vi "Plot Meas channels.vi"() -> ()   [LabVIEW 2022 SP3]
uses:
  Anemometry Sub Vis/Controls/Data for Inst Type.ctl
  Anemometry Sub Vis/Globals/Meas_global.vi
panel:
  in  "Number of Series":i32=1 min=1
  in  "Mode":T1
  in  "stop":bool
  in  "Plots":u16[](array[ring])=[4, 71, 140, 237, 267, 329, 404, 466] items=["None", "RZ (C0_P00)", "RZ (C0_P01)", "RZ (C0_P02)", "RZ (C0_P03)", "RZ (C0_P04)", "RZ (C0_P05)", "RZ (C0_P06)", "RZ (C0_P07)", "RZ (C0_P10)", "RZ (C0_P11)", "RZ (C0_P12)", "RZ (C0_P13)", "RZ (C0_P14)", "RZ (C0_P15)", "RZ (C0_P16)", "RZ (C0_P17)", "RZ (C0_P20)", "RZ (C0_P21)", "RZ (C0_P22)", "RZ (C0_P23)", "RZ (C0_P24)", "RZ (C0_P25)", "RZ (C0_P26)", "RZ (C0_P27)", "RZ (C0_P30)", "RZ (C0_P31)", "RZ (C0_P32)", "RZ (C0_P33)", "RZ (C0_P34)", "RZ (C0_P35)", "RZ (C0_P36)", "RZ (C0_P37)", "RZ (C0_P40)", "RZ (C0_P41)", "RZ (C0_P42)", "RZ (C0_P43)", "RZ (C0_P44)", "RZ (C0_P45)", "RZ (C0_P46)", "RZ (C0_P47)", "RZ (C0_P50)", "RZ (C0_P51)", "RZ (C1_P73)", "RZ (C0_P53)", "RZ (C0_P54)", "RZ (C0_P55)", "RZ (C0_P56)", "RZ (C0_P57)", "RZ (C0_P60)", "RZ (C0_P62)", "RZ (C0_P63)", "RZ (C0_P64)", "RZ (C0_P65)", "RZ (C0_P66)", "RZ (C0_P67)", "RZ (C0_P70)", "RZ (C0_P71)", "RZ (C0_P72)", "RZ (C0_P73)", "RZ (C0_P74)", "RZ (C0_P75)", "RZ (C0_P76)", "RZ (C0_P77)", "RZ (C1_P00)", "RZ (C1_P01)", "RZ (C1_P02)", "RZ (C1_P03)", "RZ (C1_P04)", "RZ (C1_P05)", "RZ (C1_P06)", "RZ (C1_P07)", "RZ (C1_P10)", "RZ (C1_P11)", "RZ (C1_P12)", "RZ (C1_P13)", "RZ (C1_P14)", "RZ (C1_P15)", "RZ (C1_P16)", "RZ (C1_P17)", "RZ (C1_P20)", "RZ (C1_P21)", "RZ (C1_P22)", "RZ (C1_P23)", "RZ (C1_P24)", "RZ (C1_P25)", "RZ (C1_P26)", "RZ (C1_P27)", "RZ (C1_P30)", "RZ (C1_P31)", "RZ (C1_P32)", "RZ (C1_P33)", "RZ (C1_P34)", "RZ (C1_P35)", "RZ (C1_P36)", "RZ (C1_P37)", "RZ (C1_P40)", "RZ (C1_P41)", "RZ (C1_P42)", "RZ (C1_P43)", "RZ (C1_P44)", "RZ (C1_P45)", "RZ (C1_P46)", "RZ (C1_P47)", "RZ (C1_P50)", "RZ (C1_P51)", "RZ (C1_P52)", "RZ (C1_P53)", "RZ (C1_P54)", "RZ (C1_P55)", "RZ (C1_P56)", "RZ (C1_P57)", "RZ (C1_P60)", "RZ (C1_P61)", "RZ (C1_P62)", "RZ (C1_P63)", "RZ (C2_P00)", "RZ (C2_P01)", "RZ (C2_P02)", "RZ (C2_P03)", "RZ (C2_P04)", "RZ (C2_P05)", "RZ (C2_P06)", "RZ (C2_P07)", "RZ (C2_P10)", "RZ (C2_P11)", "RZ (C2_P12)", "RZ (C2_P13)", "RZ (C2_P14)", "RZ (C2_P15)", "RZ (C2_P16)", "RZ (C2_P17)", "RZ (C2_P20)", "RZ (C2_P21)", "RZ (C2_P22)", "RZ (C2_P23)", "RZ (C2_P24)", "RZ (C2_P25)", "RZ (C2_P26)", "RZ (C2_P27)", "RZ (C2_P31)", "RZ (C2_P32)", "RZ (C2_P33)", "RZ (C2_P34)", "RZ (C2_P35)", "RZ (C2_P36)", "RZ (C2_P37)", "RZ (C2_P40)", "RZ (C2_P41)", "RZ (C2_P42)", "RZ (C2_P43)", "RZ (C2_P44)", "RZ (C2_P45)", "RZ (C2_P46)", "RZ (C2_P47)", "RZ (C2_P50)", "RZ (C2_P51)", "RZ (C2_P52)", "RZ (C2_P53)", "RZ (C2_P54)", "RZ (C2_P55)", "RZ (C2_P56)", "RZ (C2_P57)", "RZ (C2_P60)", "RZ (C2_P61)", "RZ (C2_P62)", "RZ (C2_P63)", "RZ (C2_P64)", "RZ (C2_P65)", "RZ (C2_P66)", "RZ (C2_P67)", "RZ (C2_P70)", "RZ (C2_P71)", "RZ (C2_P72)", "RZ (C2_P73)", "RZ (C2_P74)", "RZ (C2_P75)", "RZ (C2_P76)", "RZ (C2_P77)", "RZ (C3_P00)", "RZ (C3_P01)", "RZ (C3_P02)", "RZ (C3_P03)", "RZ (C3_P04)", "RZ (C3_P05)", "RZ (C3_P06)", "RZ (C3_P07)", "RZ (C3_P10)", "RZ (C3_P11)", "RZ (C3_P12)", "RZ (C3_P13)", "RZ (C3_P14)", "RZ (C3_P15)", "RZ (C3_P16)", "RZ (C3_P17)", "RZ (C3_P20)", "RZ (C3_P21)", "RZ (C3_P22)", "RZ (C3_P23)", "RZ (C3_P24)", "RZ (C3_P25)", "RZ (C3_P26)", "RZ (C3_P27)", "RZ (C3_P30)", "RZ (C3_P31)", "RZ (C3_P33)", "RZ (C3_P34)", "RZ (C3_P35)", "RZ (C3_P36)", "RZ (C3_P37)", "RZ (C3_P40)", "RZ (C3_P41)", "RZ (C3_P42)", "RZ (C3_P43)", "RZ (C3_P44)", "RZ (C3_P45)", "RZ (C3_P46)", "RZ (C3_P47)", "RZ (C3_P50)", "RZ (C3_P51)", "RZ (C3_P52)", "RZ (C3_P53)", "RZ (C3_P54)", "RZ (C3_P55)", "RZ (C3_P56)", "RZ (C3_P60)", "RZ (C3_P61)", "RZ (C3_P62)", "RZ (C3_P63)", "RZ (C3_P64)", "RZ (C3_P65)", "RZ (C3_P66)", "RZ (C3_P70)", "RZ (C3_P71)", "RZ (C3_P72)", "RZ (C3_P73)", "RZ (C3_P74)", "RZ (C3_P75)", "RZ (C3_P77)", "RZ (C4_P00)", "RZ (C4_P01)", "RZ (C4_P02)", "RZ (C4_P03)", "RZ (C4_P04)", "RZ (C4_P05)", "RZ (C4_P06)", "RZ (C4_P07)", "RZ (C4_P10)", "RZ (C4_P11)", "RZ (C4_P12)", "RZ (C4_P13)", "RZ (C4_P15)", "RZ (C4_P16)", "RZ (C4_P17)", "RZ (C4_P20)", "RZ (C4_P21)", "RZ (C4_P22)", "RZ (C4_P23)", "RZ (C4_P24)", "RZ (C4_P26)", "RZ (C4_P27)", "RZ (C4_P30)", "RZ (C4_P32)", "RZ (C4_P33)", "RZ (C4_P34)", "RZ (C4_P35)", "RZ (C4_P36)", "RZ (C4_P37)", "RZ (C4_P40)", "RZ (C4_P41)", "RZ (C4_P42)", "RZ (C4_P43)", "RZ (C4_P44)", "RZ (C4_P45)", "RZ (C4_P46)", "RZ (C4_P47)", "RZ (C4_P50)", "RZ (C4_P51)", "RZ (C4_P52)", "RZ (C4_P53)", "RZ (C4_P54)", "RZ (C4_P55)", "RZ (C4_P56)", "RZ (C4_P57)", "RZ (C4_P60)", "RZ (C4_P61)", "RZ (C4_P62)", "RZ (C4_P63)", "RZ (C4_P64)", "RZ (C4_P65)", "RZ (C4_P66)", "RZ (C4_P67)", "RZ (C4_P70)", "RZ (C4_P71)", "RZ (C4_P72)", "RZ (C4_P73)", "RZ (C4_P74)", "RZ (C4_P75)", "RZ (C4_P76)", "RZ (C4_P77)", "RZ (C5_P00)", "RZ (C5_P01)", "RZ (C5_P02)", "RZ (C5_P03)", "RZ (C5_P04)", "RZ (C5_P05)", "RZ (C5_P06)", "RZ (C5_P07)", "RZ (C5_P10)", "RZ (C5_P11)", "RZ (C5_P12)", "RZ (C5_P13)", "RZ (C5_P14)", "RZ (C5_P15)", "RZ (C5_P16)", "RZ (C5_P17)", "RZ (C5_P20)", "RZ (C5_P21)", "RZ (C5_P22)", "RZ (C5_P23)", "RZ (C5_P24)", "RZ (C5_P25)", "RZ (C5_P26)", "RZ (C5_P27)", "RZ (C5_P30)", "RZ (C5_P31)", "RZ (C5_P32)", "RZ (C5_P33)", "RZ (C5_P34)", "RZ (C5_P35)", "RZ (C5_P36)", "RZ (C5_P37)", "RZ (C5_P40)", "RZ (C5_P41)", "RZ (C5_P42)", "RZ (C5_P43)", "RZ (C5_P44)", "RZ (C5_P45)", "RZ (C5_P46)", "RZ (C5_P47)", "RZ (C5_P50)", "RZ (C5_P51)", "RZ (C5_P52)", "RZ (C5_P53)", "RZ (C5_P54)", "RZ (C5_P55)", "RZ (C5_P56)", "RZ (C5_P60)", "RZ (C5_P61)", "RZ (C5_P62)", "RZ (C5_P63)", "RZ (C5_P64)", "RZ (C5_P65)", "RZ (C5_P66)", "RZ (C5_P67)", "RZ (C5_P71)", "RZ (C5_P72)", "RZ (C5_P73)", "RZ (C5_P74)", "RZ (C5_P75)", "RZ (C5_P76)", "RZ (C5_P77)", "RZ (C6_P02)", "RZ (C6_P03)", "RZ (C6_P04)", "RZ (C6_P05)", "RZ (C6_P06)", "RZ (C6_P07)", "RZ (C6_P12)", "RZ (C6_P13)", "RZ (C6_P14)", "RZ (C6_P15)", "RZ (C6_P16)", "RZ (C6_P17)", "RZ (C6_P20)", "RZ (C6_P21)", "RZ (C6_P22)", "RZ (C6_P23)", "RZ (C6_P24)", "RZ (C6_P25)", "RZ (C6_P26)", "RZ (C6_P27)", "RZ (C6_P30)", "RZ (C6_P31)", "RZ (C6_P32)", "RZ (C6_P33)", "RZ (C6_P34)", "RZ (C6_P35)", "RZ (C6_P36)", "RZ (C6_P37)", "RZ (C6_P40)", "RZ (C6_P41)", "RZ (C6_P42)", "RZ (C6_P43)", "RZ (C6_P44)", "RZ (C6_P45)", "RZ (C6_P46)", "RZ (C6_P47)", "RZ (C6_P50)", "RZ (C6_P51)", "RZ (C6_P52)", "RZ (C6_P53)", "RZ (C6_P54)", "RZ (C6_P55)", "RZ (C6_P56)", "RZ (C6_P60)", "RZ (C6_P61)", "RZ (C6_P62)", "RZ (C6_P63)", "RZ (C6_P64)", "RZ (C6_P65)", "RZ (C6_P66)", "RZ (C6_P67)", "RZ (C6_P70)", "RZ (C6_P71)", "RZ (C6_P72)", "RZ (C6_P73)", "RZ (C6_P74)", "RZ (C6_P75)", "RZ (C6_P76)", "RZ (C6_P77)", "RZ (C7_P00)", "RZ (C7_P01)", "RZ (C7_P02)", "RZ (C7_P03)", "RZ (C7_P04)", "RZ (C7_P05)", "RZ (C7_P06)", "RZ (C7_P07)", "RZ (C7_P10)", "RZ (C7_P11)", "RZ (C7_P12)", "RZ (C7_P13)", "RZ (C7_P14)", "RZ (C7_P15)", "RZ (C7_P16)", "RZ (C7_P17)", "RZ (C7_P20)", "RZ (C7_P21)", "RZ (C7_P22)", "RZ (C7_P23)", "RZ (C7_P24)", "RZ (C7_P25)", "RZ (C7_P26)", "RZ (C7_P27)", "RZ (C7_P30)", "RZ (C7_P31)", "RZ (C7_P32)", "RZ (C7_P33)", "RZ (C7_P34)", "RZ (C7_P35)", "RZ (C7_P36)", "RZ (C7_P37)", "RZ (C7_P40)", "RZ (C7_P41)", "RZ (C7_P42)", "RZ (C7_P43)", "RZ (C7_P44)", "RZ (C7_P45)", "RZ (C7_P46)", "RZ (C7_P47)", "RZ (C7_P50)", "RZ (C7_P51)", "RZ (C7_P52)", "RZ (C7_P53)", "RZ (C7_P54)", "RZ (C7_P55)", "RZ (C7_P56)", "RZ (C7_P57)", "RZ (C7_P60)", "RZ (C7_P61)", "RZ (C7_P62)", "RZ (C7_P63)", "RZ (C7_P64)", "RZ (C7_P65)", "RZ (C7_P66)", "RZ (C7_P67)", "RZ (C7_P70)", "RZ (C7_P71)", "RZ (C7_P72)", "RZ (C7_P73)", "RZ (C7_P74)", "RZ (C7_P75)", "RZ (C7_P76)", "RZ (C7_P77)", "FF (C)", "FF (Cref)"]
  out "XY Graph":cluster{"Time (s)":dbl[], "Eng Values":dbl[]}[](graph)
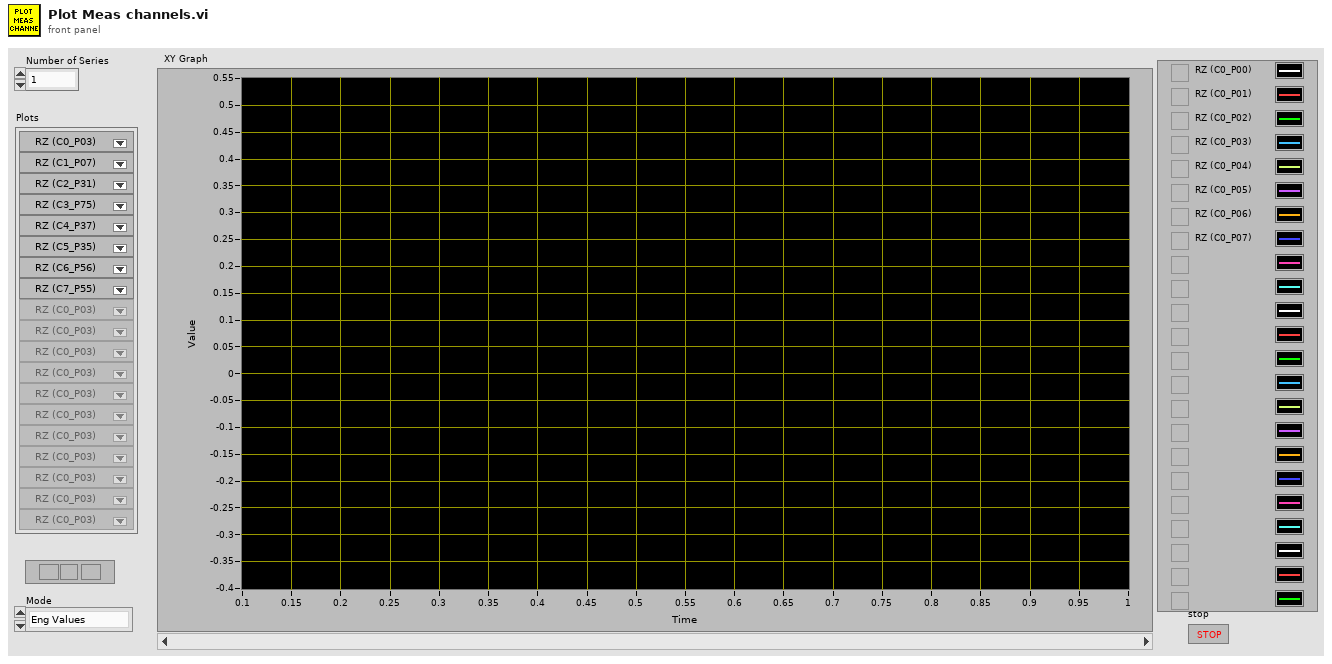
[diagram p1: front panel]
types:
  T1 = typedef "Data for Inst Type.ctl" = enum16{"Eng Values", "Voltage"}
  T2 = typedef "Analysis_info_cluster.ctl" = cluster{"Colour":u32, "Inst type":T3, "Inst name":string, "Symbol":string, "Code name":string, "Extra Info":string, "Inst Array":T4, "Extra Titles":string[], "Extra Values":string[], "U":dbl, "u^2":dbl, "u^3":dbl, "u^4":dbl, "Skew_u":dbl, "Kurt_u":dbl, "Sd Error in Mean":dbl, "% u'/U":dbl, "X":dbl, "Y":dbl, "Z":dbl, "Timescale integral Estimate":dbl, "Sd Error in Variance":dbl, "Calib File":path, "Calib Constants":dbl[], "Output Position":bool, "Stats":enum16{"None", "Basic", "Full"}, "Av Sampling Rate":dbl, "Av No of Samples":dbl, "Total Meas Time (s)":dbl, "ADAM Ch Name":string, "Max value":dbl, "Min value":dbl, "Req Sample Rate Hz":dbl, "Sync Delay Time (s)":dbl, "Ch No":i16, "Device":string, "Use Latest Calib":bool, "Port":string, "Metadata Ch Names":string[], "Metadata Ch Values":string[], "Label":string}
  T3 = typedef "Inst_type.ctl" = enum16{"Raw voltage", "Raw with zero offsetting", "Propeller anemometer", "Pressure Transducer", "Pitot-static tube", "Hot wire", "Cross wire 1", "Cross wire 2", "Generic Linear", "Generic Polynomial", "Generic BackPoly", "Fast FID", "Thermocouple", "Cold wire", "Pulsed Wire", "LDA Vel", "LDA Tran time", "LDA Arr time", "Microphone"}
  T4 = typedef "Instrument_Array.ctl" = enum16{"PWA", "LDA", "Analogue"}
  T5 = typedef "Time_Trace_Cluster.ctl" = cluster{"Weighting":dbl[], "Voltage":dbl[], "Eng Values":dbl[]}
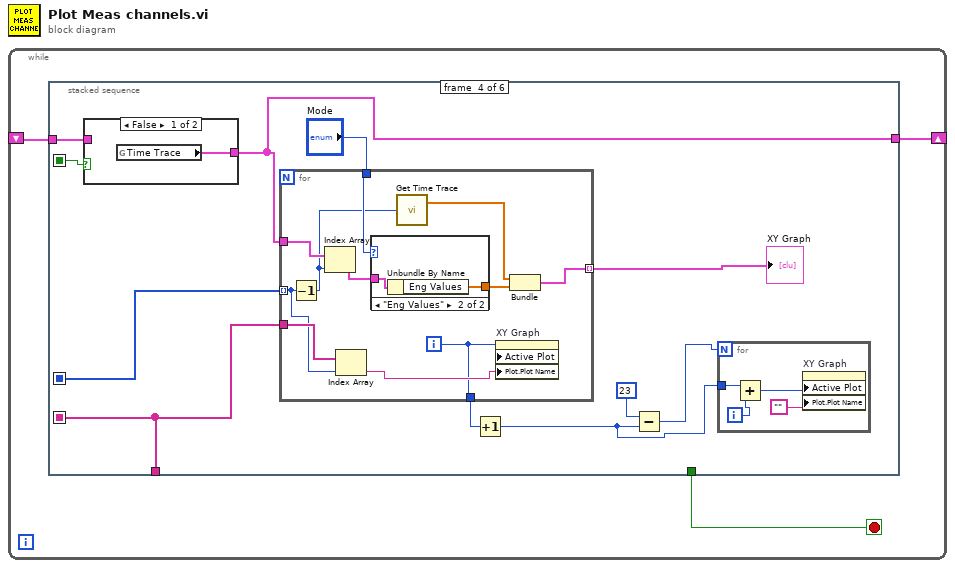
[diagram p0: block diagram]
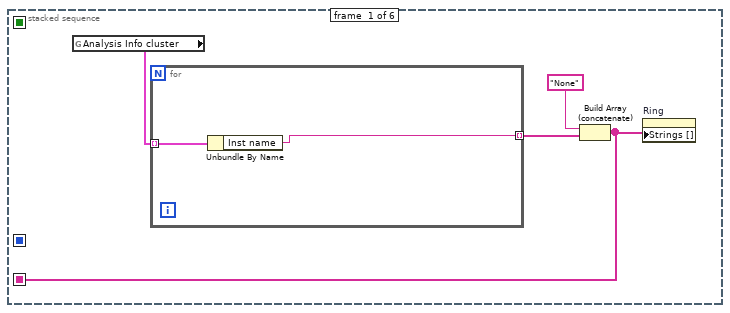
[diagram p2: hidden frame]
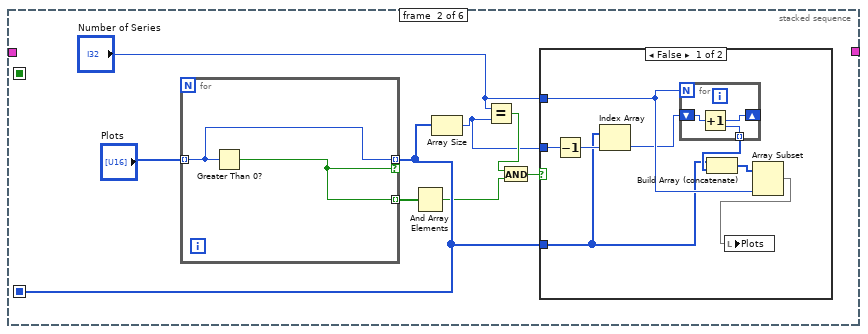
[diagram p3: hidden frame]
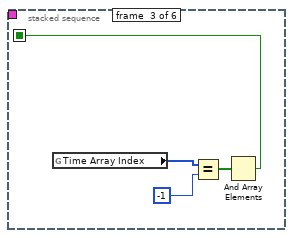
[diagram p5: hidden frame]
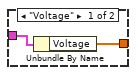
[diagram p7: hidden frame]
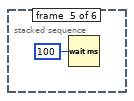
[diagram p8: hidden frame]
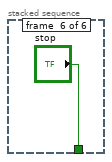
[diagram p9: hidden frame]
diagram:
  n1 = while {
    shift-right: [w2] -> _
    shift-left: _ -> [w1]
    stop <- w3 stop-if-true
    n2 = stacked-sequence {
      seq-local: [_ w15 _ _ _ _] -> [_ _ _ w43 _ _]
      seq-local: [w4 _ _ _ _ _] -> [_ _ _ w38 _ _]
      seq-local: [_ _ w30 _ _ _] -> [_ _ _ w36 _ _]
      tunnel: [_ _ _ w38 _ _] -> _
      tunnel: [_ _ _ _ _ "stop"] -> w3
      tunnel: [_ _ _ w35 _ _] -> w2
      tunnel: w1 -> [_ _ _ w34 _ _]
      frame #0 {
        n3 = global read "Meas_global.vi" "Analysis Info cluster"() -> (w5:T2[])
        n4 = for {
          tunnel: w5 -> [w9] mode=indexing
          tunnel: [w8] -> w7 mode=indexing
          n5 = Unbundle By Name(w9) -> ("Inst name"=w8:string)
        }
        n6 = Build Array (concatenate)("None", w7) -> (w4:string[])
        n7 = property on="Ring" class="Ring (strict)"("Strings []"=w4) -> ()  [unwired: 2 in, 2 out]
      }
      frame #1 {
        n8 = for {
          tunnel: "Plots" -> [w29] mode=indexing
          tunnel: [w29] -> w15 mode=indexing if=w28
          tunnel: [w28] -> w16 mode=indexing
          n9 = Greater Than 0?(x=w29) -> (x > 0?=w28:bool)
        }
        n10 = And Array Elements(Boolean array=w16) -> (logical AND=w13:bool)
        n11 = Array Size(array=w15) -> (size(s)=w10:i32)
        n12 = Equal?(x="Number of Series", y=w10) -> (x = y?=w14:bool)
        n13 = And(x=w14, y=w13) -> (x .and. y?=w12:bool)
        n14 = case shown="False" w12 {
          tunnel: w15 -> [w19 _]
          tunnel: "Number of Series" -> [w22 _]
          tunnel: w10 -> [w21 _]
          frame False {
            n15 = Decrement(x=w21) -> (x-1=w20:i32)
            n16 = Index Array(array=w19, index=w20) -> (element=w18:u16)
            n17 = for {
              N: w22 -> [_]
              tunnel: [w26] -> w23 mode=indexing
              shift-right: [w26] -> _
              shift-left: w18 -> [w27]
              n18 = Increment(x=w27) -> (x+1=w26:u16)
            }
            n19 = Build Array (concatenate)(w19, w23) -> (w25:u16[])
            n20 = Array Subset(array=w25, length=w22) -> (w24:u16[])  [unwired: 1 in]
            n21 = local write "Plots"(w24) -> ()
          }
          frame True {
          }
        }
      }
      frame #2 {
        n22 = global read "Meas_global.vi" "Time Array Index"() -> (w32:i32[])
        n23 = Equal?(x=w32, y=-1) -> (x = y?=w31:bool[])
        n24 = And Array Elements(Boolean array=w31) -> (logical AND=w30:bool)
      }
      frame #3 {
        n25 = case shown="False" w36 {
          tunnel: [w45 w46] -> w35
          tunnel: w34 -> [_ w46]
          frame False {
            n26 = global read "Meas_global.vi" "Time Trace"() -> (w45:T5[])
          }
          frame True {
          }
        }
        n27 = for {
          tunnel: w35 -> [w61]
          tunnel: [w59] -> w44 mode=indexing
          tunnel: w43 -> [w54] mode=indexing
          tunnel: w38 -> [w57]
          tunnel: [w55] -> w40
          tunnel: "Mode" -> [w53]
          i -> [w55]
          n28 = Decrement(x=w54) -> (x-1=w52:u16)
          n29 = Index Array(array=w61, index=w52) -> (element=w60:T5)
          n30 = Index Array(array=w57, index=w54) -> (element=w56:string)
          n31 = case shown="\"Eng Values\"" w53 {
            tunnel: w60 -> [w63 w65]
            tunnel: [w62 w64] -> w58
            frame "Voltage" {
              n32 = Unbundle By Name(w63) -> ("Voltage"=w62:dbl[])
            }
            frame "Eng Values" {
              n33 = Unbundle By Name(w65) -> ("Eng Values"=w64:dbl[])
            }
          }
          n34 = call "Get Time Trace.vi"("Channel Index"=w52) -> ("Time (s)"=w51:dbl[])  [unwired: 1 out]
          n35 = property on="XY Graph" class="XYGraph (strict)"("Active Plot"=w55, "Plot.Plot Name"=w56) -> ()  [unwired: 2 in, 2 out]
          n36 = Bundle("Time (s)"=w51, "Eng Values"=w58) -> (w59:cluster{"Time (s)":dbl[], "Eng Values":dbl[]})  [unwired: 1 in]
        }
        "XY Graph" <- w44
        n37 = Increment(x=w40) -> (x+1=w39:i32)
        n38 = Subtract(x=23, y=w39) -> (x-y=w41:i32)
        n39 = for {
          N: w41 -> [_]
          tunnel: w39 -> [w49]
          i -> [w50]
          n40 = Add(x=w49, y=w50) -> (x+y=w48:i32)
          n41 = property on="XY Graph" class="XYGraph (strict)"("Active Plot"=w48, "Plot.Plot Name"="") -> ()  [unwired: 2 in, 2 out]
        }
      }
      frame #4 {
        n42 = Wait (ms)(milliseconds to wait=u32 100) -> ()  [unwired: 1 out]
      }
      frame #5 {
      }
    }
  }
